vi "mks946_sub_get_dbl.vi"(6 "error in (no error)":errorcluster, 7 "VISA_ref_in":refnum<visa-resource-name>="COM3", 10 "command":string="PR", 11 "address":i32) -> (0 "status":bool, 2 "message":string, 3 "value":dbl, 4 "error out":errorcluster={"status"=TRUE, "code"=1, "source"="Scan From String (arg 1) in mks946_sub_get.vi"}, 5 "VISA_ref_out":refnum<visa-resource-name>="COM3")   [LabVIEW 2019]
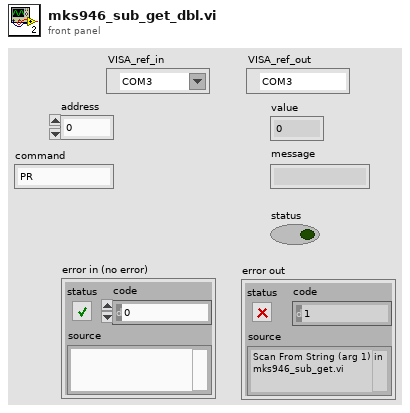
[diagram p1: front panel]
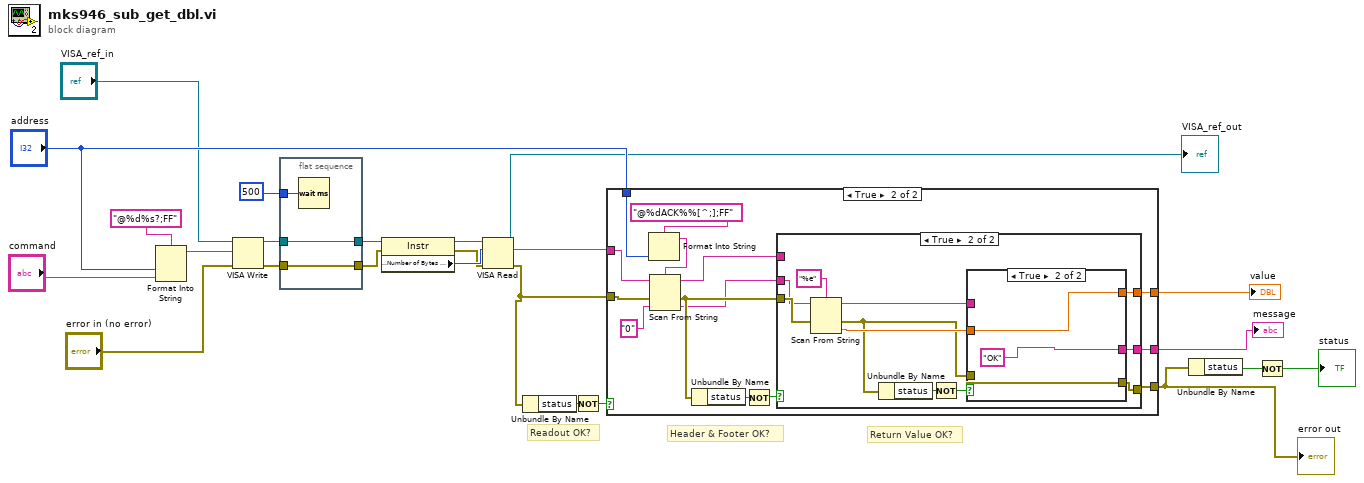
[diagram p0: block diagram]
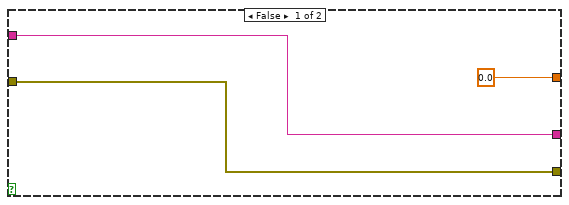
[diagram p2: hidden frame]
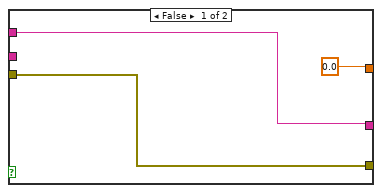
[diagram p3: hidden frame]
diagram:
  # "Return Value OK?"
  # "Header & Footer OK?"
  # "Readout OK?"
  n1 = Format Into String(format string="@%d%s?;FF", "address", "command") -> (resulting string=w8:string)  [unwired: 2 in, 1 out]
  n2 = VISA Write(VISA resource name="VISA_ref_in", write buffer=w8, error in (no error)="error in (no error)") -> (VISA resource name out=w4:refnum<visa-resource-name>, error out=w3:errorcluster)  [unwired: 1 out]
  n3 = flat-sequence {
    tunnel: w3 -> [w26]
    tunnel: [w26] -> w13
    tunnel: w4 -> [w25]
    tunnel: [w25] -> w12
    tunnel: u32 500 ("mks946_delay") -> [w27]
    frame #0 {
      n4 = Wait (ms)(milliseconds to wait=w27) -> ()  [unwired: 1 out]
    }
  }
  n5 = property class="Instr"(reference=w12, error in=w13) -> (reference out=w21:refnum<visa-resource-name>, error out=w22:errorcluster, "Serial Settings:Number of Bytes at Serial Port"=w23:u32)
  n6 = VISA Read(VISA resource name=w21, byte count=w23, error in (no error)=w22) -> (VISA resource name out=→"VISA_ref_out":refnum<visa-resource-name>, read buffer=w15:string, error out=w16:errorcluster)  [unwired: 1 out]
  n7 = Unbundle By Name(w16) -> ("status"=w11:bool)
  n8 = Not(x=w11) -> (.not. x?=w14:bool)
  n9 = case shown="True" w14 {
    tunnel: [w30 w35] -> w19
    tunnel: w15 -> [w29 w44]
    tunnel: w16 -> [w30 w43]
    tunnel: "address" -> [_ w42]
    tunnel: [w29 w32] -> w2
    tunnel: [0.0 w31] -> w1
    frame False {
    }
    frame True {
      n10 = Format Into String(format string="@%dACK%%[^;];FF", w42) -> (resulting string=w41:string)  [unwired: 2 in, 1 out]
      n11 = Scan From String(format string=w41, input string=w44, error in=w43, default 1="0") -> (remaining string=w34:string, error out=w37:errorcluster, output 1=w36:string)  [unwired: 1 in, 1 out]
      n12 = Unbundle By Name(w37) -> ("status"=w39:bool)
      n13 = Not(x=w39) -> (.not. x?=w38:bool)
      n14 = case shown="True" w38 {
        tunnel: w37 -> [w47 w57]
        tunnel: w36 -> [_ w56]
        tunnel: [w47 w51] -> w35
        tunnel: w34 -> [w46 _]
        tunnel: [w46 w49] -> w32
        tunnel: [0.0 w48] -> w31
        frame False {
        }
        frame True {
          n15 = Scan From String(format string="%e", input string=w56, error in=w57) -> (remaining string=w50:string, error out=w52:errorcluster, output 1=w54:dbl)  [unwired: 2 in, 1 out]
          n16 = Unbundle By Name(w52) -> ("status"=w55:bool)
          n17 = Not(x=w55) -> (.not. x?=w53:bool)
          n18 = case shown="True" w53 {
            tunnel: w54 -> [w59 w62]
            tunnel: w52 -> [w61 w64]
            tunnel: [w61 w64] -> w51
            tunnel: w50 -> [w60 _]
            tunnel: [w60 "OK"] -> w49
            tunnel: [w59 w62] -> w48
            frame False {
            }
            frame True {
            }
          }
        }
      }
    }
  }
  "error out" <- w19
  "value" <- w1
  "message" <- w2
  n19 = Unbundle By Name(w19) -> ("status"=w17:bool)
  n20 = Not(x=w17) -> (.not. x?=→"status":bool)
